vi "Set dome.vi"(2 "Dome In":dbl format="%.2f") -> (0 "DONE":bool, 1 "Dome Out":dbl format="%.2f")   [LabVIEW 2011]
panel:
  in  "Bouton Annuler":bool
  in  "OK":bool
  in  "Coupole":dbl=1.2 min=1.0 max=360.0 step=1.0
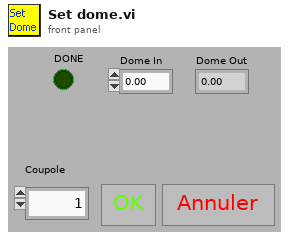
[diagram p1: front panel]
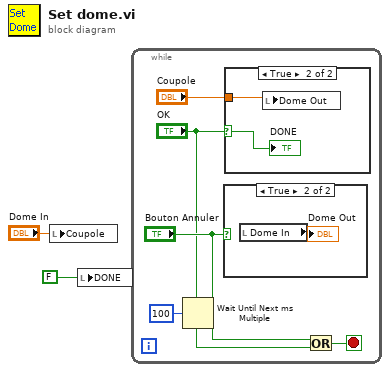
[diagram p0: block diagram]
diagram:
  n1 = local write "Coupole"("Dome In") -> ()
  n2 = local write "DONE"(FALSE) -> ()
  n3 = while {
    stop <- w5 stop-if-true
    n4 = Wait Until Next ms Multiple(millisecond multiple=u32 100 ("n millisecondes")) -> ()  [unwired: 1 out]
    n5 = case shown="True" "Bouton Annuler" {
      frame False {
      }
      frame True {
        n6 = local read "Dome In"() -> (→"Dome Out":dbl)
      }
    }
    n7 = case shown="True" "OK" {
      selector: "OK" -> [_ w9]
      tunnel: "Coupole" -> [_ w10]
      frame False {
      }
      frame True {
        n8 = local write "Dome Out"(w10) -> ()
        "DONE" <- w9
      }
    }
    n9 = Or(x="Bouton Annuler", y="OK") -> (x .or. y?=w5:bool)
  }
